vi "Ring plots update.vi"(10 "New Plots":cluster{"X":u16, "Y":u16}[](array[cluster]) {"Y" items=["Select channel...", "Time", "Y"]; "X" items=["Select channel...", "Time", "Y"]}, 11 "Old Plots":cluster{"X":u16, "Y":u16}[](array[cluster]) {"Y" items=["Select channel...", "Time", "Y"]; "X" items=["Select channel...", "Time", "Y"]}) -> (3 "Plots":cluster{"X":u16, "Y":u16}[](array[cluster]) {"Y" items=["Select channel...", "Time", "Y"]; "X" items=["Select channel...", "Time", "Y"]}, 5 "Replot?":bool)   [LabVIEW 2019]
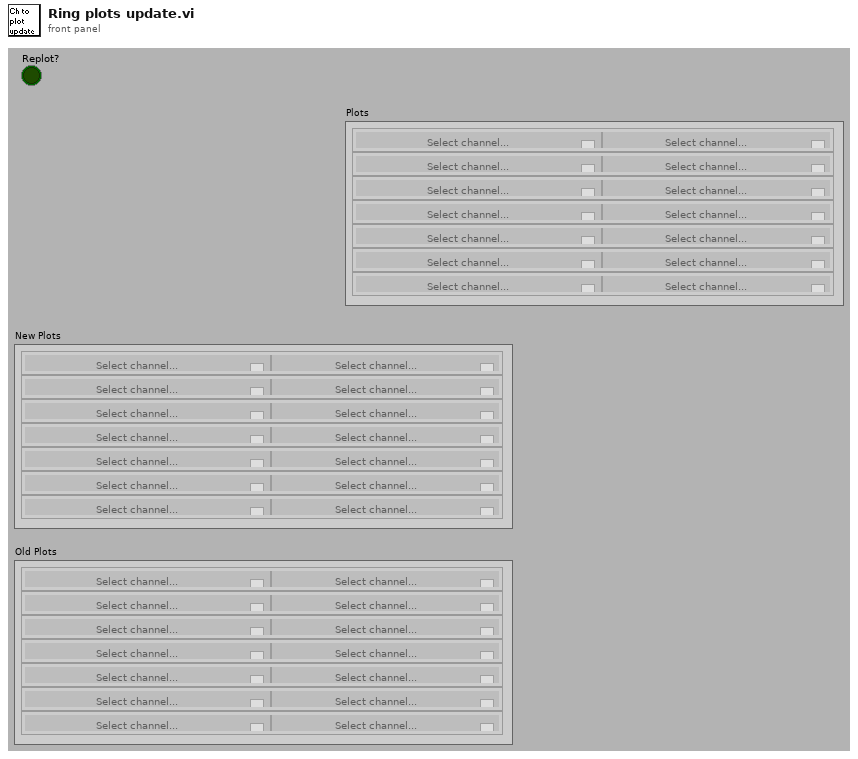
[diagram p1: front panel]
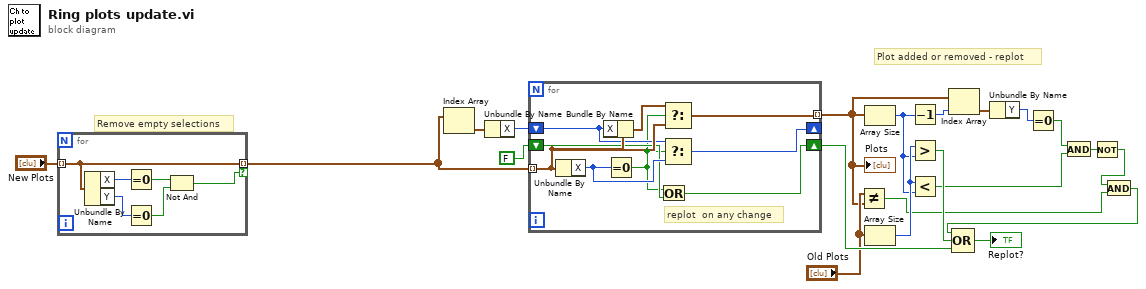
[diagram p0: block diagram]
diagram:
  # "Plot added or removed - replot"
  # "Remove empty selections"
  n1 = for {
    tunnel: "New Plots" -> [w25] mode=indexing
    tunnel: [w25] -> w12 mode=indexing if=w22
    n2 = Unbundle By Name(w25) -> ("X"=w27:u16, "Y"=w26:u16)
    n3 = Equal To 0?(x=w27) -> (x = 0?=w24:bool)
    n4 = Equal To 0?(x=w26) -> (x = 0?=w23:bool)
    n5 = Not And(1:w23, 2:w24) -> (0:w22:bool)
  }
  n6 = Index Array(array=w12) -> (element=w20:cluster{"X":u16, "Y":u16})  [unwired: 1 in]
  n7 = Unbundle By Name(w20) -> ("X"=w19:u16)
  n8 = for {
    tunnel: w12 -> [w35] mode=indexing
    shift-right: [w32] -> _
    shift-left: w19 -> [w33]
    tunnel: [w31] -> w8 mode=indexing
    shift-right: [w28] -> w16
    shift-left: FALSE -> [w30]
    # "replot  on any change"
    n9 = Unbundle By Name(w35) -> ("X"=w34:u16)
    n10 = Bundle By Name(cluster=w35, "X"=w33) -> (w36:cluster{"X":u16, "Y":u16})
    n11 = Equal To 0?(x=w34) -> (x = 0?=w29:bool)
    n12 = Or(x=w29, y=w30) -> (x .or. y?=w28:bool)
    n13 = Select(t=w36, s=w29, f=w35) -> (s? t:f=w31:cluster{"X":u16, "Y":u16})
    n14 = Select(t=w33, s=w29, f=w34) -> (s? t:f=w32:u16)
  }
  "Plots" <- w8
  n15 = Not Equal?(x="Old Plots", y=w8) -> (x != y?=w2:bool)
  n16 = Array Size(array=w8) -> (size(s)=w11:i32)
  n17 = Array Size(array="Old Plots") -> (size(s)=w13:i32)
  n18 = Decrement(x=w11) -> (x-1=w10:i32)
  n19 = Greater?(x=w13, y=w11) -> (0:w17:bool)
  n20 = Less?(x=w13, y=w11) -> (x < y?=w5:bool)
  n21 = Index Array(array=w8, index=w10) -> (element=w9:cluster{"X":u16, "Y":u16})
  n22 = Unbundle By Name(w9) -> ("Y"=w7:u16)
  n23 = Equal To 0?(x=w7) -> (x = 0?=w6:bool)
  n24 = And(x=w6, y=w5) -> (x .and. y?=w4:bool)
  n25 = Not(x=w4) -> (.not. x?=w3:bool)
  n26 = And(x=w3, y=w2) -> (x .and. y?=w1:bool)
  n27 = Compound Arithmetic op=OR(w1, w17, w16) -> (→"Replot?":bool)
